vi "Move Down Waveform in List.vi"(7 "Waveform List Ctl Ref":refnum<vi>, 8 "error in (no error)":errorcluster, 11 "Canvas Wfm Array In":waveform(dbl)[](array[waveform])) -> (0 "error out":errorcluster, 3 "Canvas Wfm Array Out":waveform(dbl)[](array[waveform]))   [LabVIEW 2025, in "TDMS Waveform Creator UI.lvlib"]
uses:
  TDMS Waveform Creator UI.lvlib
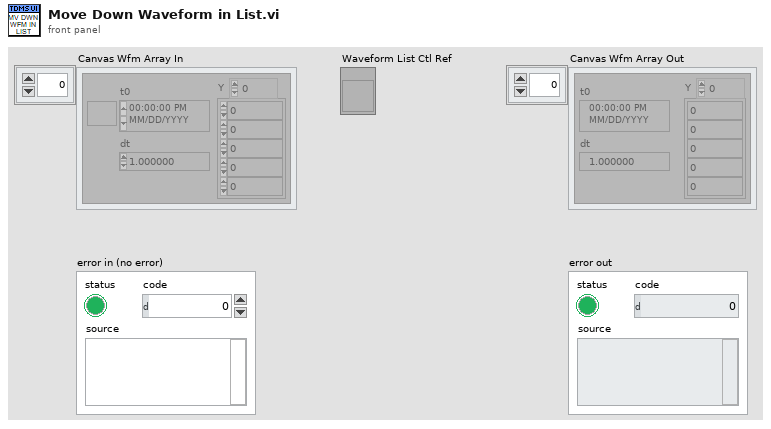
[diagram p1: front panel]
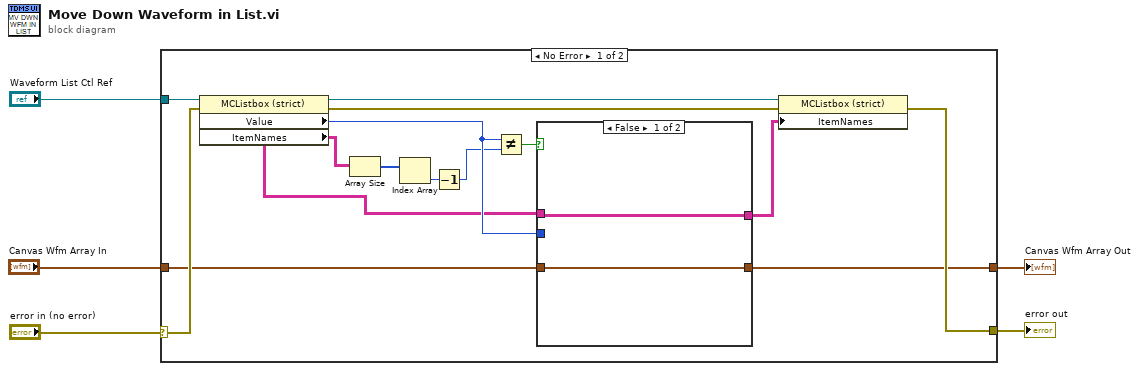
[diagram p0: block diagram]
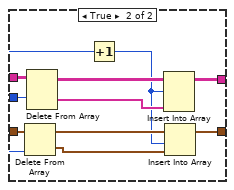
[diagram p2: hidden frame]
diagram:
  n1 = case shown="No Error" "error in (no error)" {
    selector: "error in (no error)" -> [w17 w33]
    tunnel: "Waveform List Ctl Ref" -> [w19 _]
    tunnel: "Canvas Wfm Array In" -> [w14 w32]
    tunnel: [w12 w32] -> w2
    tunnel: [w16 w33] -> w1
    frame No Error {
      n2 = property class="MCListbox (strict)"(reference=w19, error in=w17) -> (reference out=w18:refnum<vi>, error out=w15:errorcluster, "Value"=w11:i32, "ItemNames"=w10:string[][])
      n3 = Array Size(array=w10) -> (size(s)=w9:i32[])
      n4 = Index Array(array=w9) -> (element=w8:i32)  [unwired: 1 in]
      n5 = Decrement(x=w8) -> (x-1=w7:i32)
      n6 = Not Equal?(x=w11, y=w7) -> (x != y?=w6:bool)
      n7 = case shown="False" w6 {
        tunnel: w14 -> [w20 w29]
        tunnel: [w21 w28] -> w13
        tunnel: [w20 w26] -> w12
        tunnel: w11 -> [_ w23]
        tunnel: w10 -> [w21 w22]
        frame False {
        }
        frame True {
          n8 = Delete From Array(array=w29, index=w23) -> (deleted portion=w25:waveform(dbl), array with subset deleted=w31:waveform(dbl)[])  [unwired: 1 in]
          n9 = Delete From Array(array=w22, index (row)=w23) -> (deleted portion=w27:string[], array with subset deleted=w30:string[][])  [unwired: 2 in]
          n10 = Increment(x=w23) -> (x+1=w24:i32)
          n11 = Insert Into Array(array=w30, index (row)=w24, new element=w27) -> (w28:string[][])  [unwired: 1 in]
          n12 = Insert Into Array(array=w31, index=w24, new element=w25) -> (w26:waveform(dbl)[])
        }
      }
      n13 = property class="MCListbox (strict)"(reference=w18, error in=w15, "ItemNames"=w13) -> (error out=w16:errorcluster)  [unwired: 1 out]
    }
    frame Error {
    }
  }
  "error out" <- w1
  "Canvas Wfm Array Out" <- w2
